vi "U64 Millisecond Tick Count.vi"(8 "Error In":errorcluster) -> (0 "Error Out":errorcluster, 2 "U64 millisecond \ntimer value":u64 caption="U64 millisecond timer value")   [LabVIEW 2013, in "FindName Task_Manager.lvlib"]
doc: "Returns the value of the millisecond timer, as a U64. This tick count will wrap every 584 million years, as opposed to the native U32 variation which will wrap every 49.7 days. Any error in is passed through to error out, but the this VI ignores error in and will perform its function regqardless.\n\nBe careful to mind your data types when using the U64, as any inadvertent coercion to another data type could eliminate this extra precision."
uses:
  FindName Task_Manager.lvlib
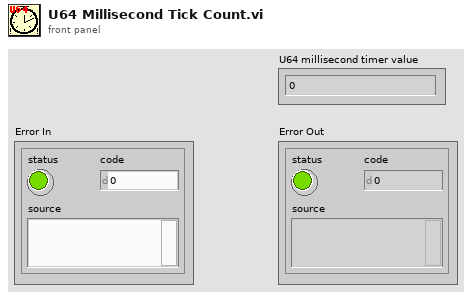
[diagram p1: front panel]
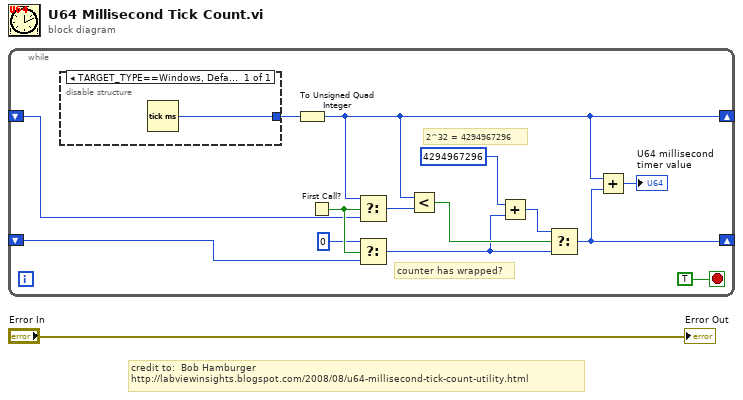
[diagram p0: block diagram]
diagram:
  # "credit to:  Bob Hamburger\nhttp://labviewinsights.blogspot.com/2008/08/u64-millisecond-tick-count-utility.html"
  n1 = while {
    shift-right: [w12] -> _
    shift-left: _ -> [w11]
    shift-right: [w6] -> _
    shift-left: _ -> [w9]
    stop <- TRUE stop-if-true
    # "counter has wrapped?"
    # "2^32 = 4294967296"
    n2 = disable-structure shown="TARGET_TYPE==Windows, Default" {
      disable-tunnel: [w16] -> w15
      frame condition #0 (active) {
        n3 = Tick Count (ms)() -> (millisecond timer value=w16:u32)
      }
    }
    n4 = To Unsigned Quad Integer(1:w15) -> (0:w12:u64)
    n5 = First Call?() -> (First Call?: T/F=w13:bool)
    n6 = Select(t=w12, s=w13, f=w11) -> (s? t:f=w8:u64)
    n7 = Select(t=u64 0, s=w13, f=w9) -> (s? t:f=w4:u64)
    n8 = Less?(x=w12, y=w8) -> (x < y?=w7:bool)
    n9 = Add(x=u64 4294967296, y=w4) -> (x+y=w3:u64)
    n10 = Select(t=w3, s=w7, f=w4) -> (s? t:f=w6:u64)
    n11 = Add(x=w12, y=w6) -> (x+y=→"U64 millisecond \ntimer value":u64)
  }
  "Error Out" <- "Error In"
